vi "test3-SyncMessage_API.vi"(8 "error in (no error)":errorcluster, 11 "TestCase in":refnum<class "testcase-CSMMessage.lvclass">) -> (0 "error out":errorcluster, 3 "TestCase out":refnum<class "testcase-CSMMessage.lvclass">)   [LabVIEW 2017, in "testcase-CSMMessage.lvclass"]
uses:
  testcase-CSMMessage.lvclass
  31aab9b4-27f2-4601-9b9c-9d12425ab602.vi
  src/user.lib/_NEVSTOP/Communicable State Machine(CSM)/AdvanceAPI/CSM - Make String Arguments Safe.vi
  src/user.lib/_NEVSTOP/Communicable State Machine(CSM)/AdvanceAPI/CSM - Keywords.vi
  <vilib>/addons/_JKI Toolkits/VI Tester/TestCase.llb/TestCase.lvclass
  src/user.lib/_NEVSTOP/Communicable State Machine(CSM)/Communicable State Machine.lvlib
  C:/Program Files (x86)/National Instruments/LabVIEW 2017/vi.lib/addons/_JKI Toolkits/VI Tester/TestCase.llb/TestCase.lvclass
panel:
  out "Attribute":T1(array[cluster])
  out "Found":bool[](array[boolean])
  out "Loopcount":i32
  out "concatenated string":string
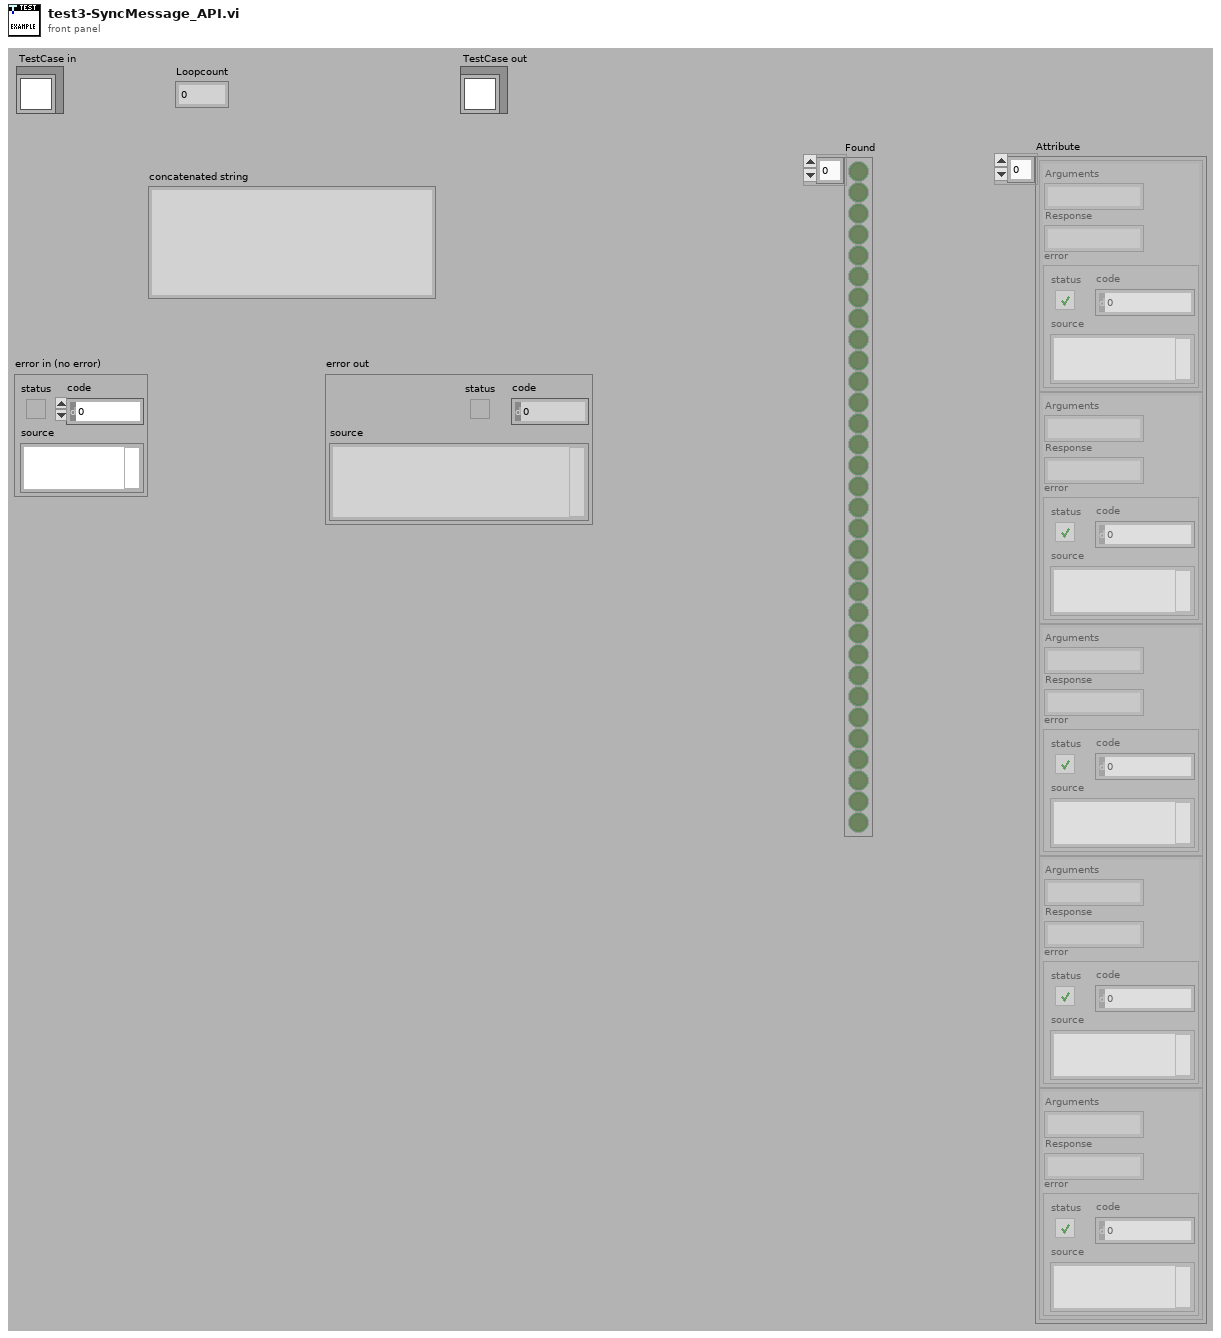
[diagram p1: front panel]
types:
  T1 = cluster{"Arguments":string, "Response":string, "error":errorcluster}[]
  T2 = cluster{"Arguments":string, "Response":string, "error":errorcluster}
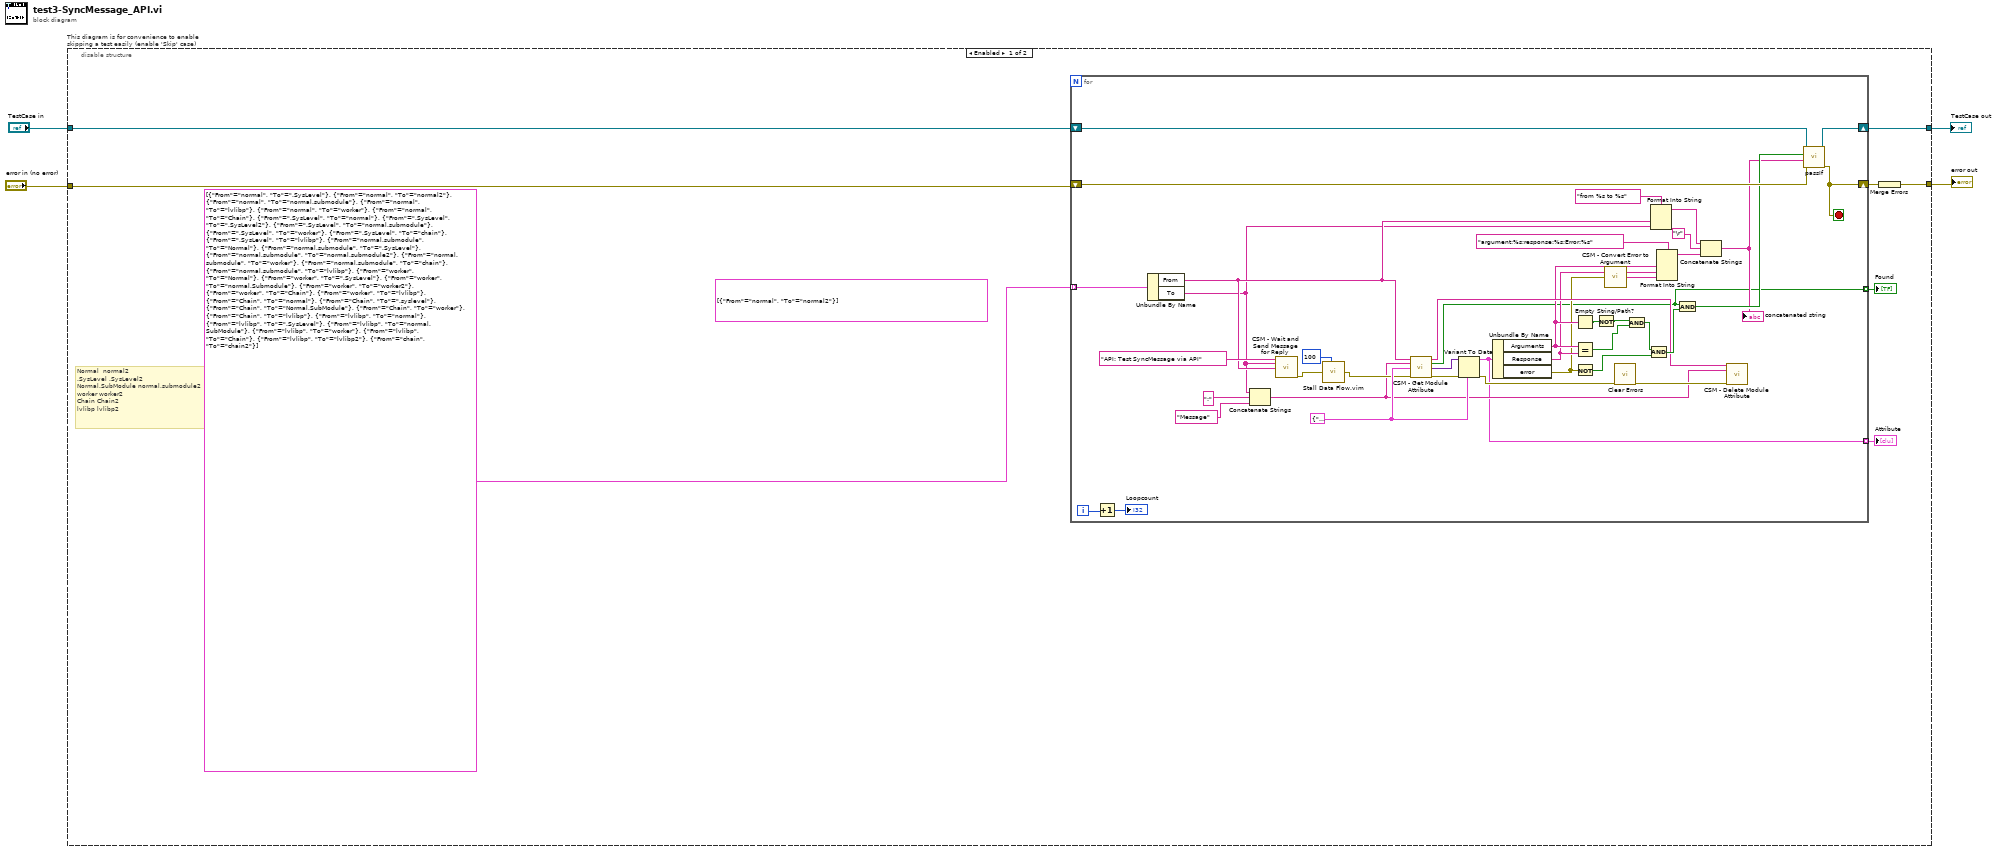
[diagram p0: block diagram]
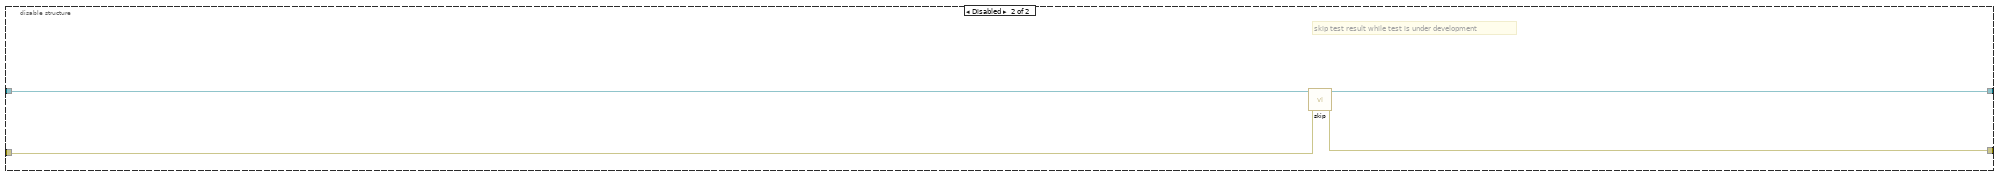
[diagram p2: hidden frame]
diagram:
  n1 = disable-structure "This diagram is for convenience to enable skipping a test easily (enable 'Skip' case)" shown="Enabled" {
    disable-tunnel: "TestCase in" -> [w12 w57]
    disable-tunnel: [w11 w55] -> w1
    disable-tunnel: [w8 w56] -> w3
    disable-tunnel: "error in (no error)" -> [w9 w54]
    frame Enabled {
      (unwired) cluster{"From":string, "To":string}[] [{"From"="normal", "To"="normal2"}]
      # "Normal  normal2\n.SysLevel .SysLevel2\nNormal.SubModule normal.submodule2\nworker worker2\nChain Chain2\nlvlibp lvlibp2"
      n2 = for {
        tunnel: cluster{"From":string, "To":string}[] [{"From"="normal", "To"=".SysLevel"}, {"From"="normal", "To"="normal2"}, {"From"="normal", "To"="normal.submodule"}, {"From"="normal", "To"="lvlibp"}, {"From"="normal", "To"="worker"}, {"From"="normal", "To"="Chain"}, {"From"=".SysLevel", "To"="normal"}, {"From"=".SysLevel", "To"=".SysLevel2"}, {"From"=".SysLevel", "To"="normal.submodule"}, {"From"=".SysLevel", "To"="worker"}, {"From"=".SysLevel", "To"="chain"}, {"From"=".SysLevel", "To"="lvlibp"}, {"From"="normal.submodule", "To"="Normal"}, {"From"="normal.submodule", "To"=".SysLevel"}, {"From"="normal.submodule", "To"="normal.submodule2"}, {"From"="normal.submodule", "To"="worker"}, {"From"="normal.submodule", "To"="chain"}, {"From"="normal.submodule", "To"="lvlibp"}, {"From"="worker", "To"="Normal"}, {"From"="worker", "To"=".SysLevel"}, {"From"="worker", "To"="normal.Submodule"}, {"From"="worker", "To"="worker2"}, {"From"="worker", "To"="Chain"}, {"From"="worker", "To"="lvlibp"}, {"From"="Chain", "To"="normal"}, {"From"="Chain", "To"=".syslevel"}, {"From"="Chain", "To"="Normal.SubModule"}, {"From"="Chain", "To"="worker"}, {"From"="Chain", "To"="lvlibp"}, {"From"="lvlibp", "To"="normal"}, {"From"="lvlibp", "To"=".SysLevel"}, {"From"="lvlibp", "To"="normal.SubModule"}, {"From"="lvlibp", "To"="worker"}, {"From"="lvlibp", "To"="Chain"}, {"From"="lvlibp", "To"="lvlibp2"}, {"From"="chain", "To"="chain2"}] -> [w44] mode=indexing
        shift-right: [w52] -> w11
        shift-left: w12 -> [w53]
        shift-right: [w25] -> w10
        shift-left: w9 -> [w51]
        tunnel: [w16] -> w6 mode=indexing
        tunnel: [w15] -> w5 mode=indexing
        i -> [w18]
        stop <- w25 stop-if-true
        w48 = T2 {"Arguments"="", "Response"="", "error"={"status"=FALSE, "code"=0, "source"=""}}
        n3 = Increment(x=w18) -> (x+1=→"Loopcount":i32)
        n4 = Unbundle By Name(w44) -> ("From"=w22:string, "To"=w20:string)
        n5 = Concatenate Strings(w20, ":" ("string"), "Message" ("string")) -> (w21:string)
        n6 = call "CSM - Wait and Send Message for Reply.vi"("State"="API: Test SyncMessage via API", "Arguments (\"\")"=w20, "Target Module"=w22) -> ("error out"=w14:errorcluster)  [unwired: 9 in, 3 out]
        n7 = call "Stall Data Flow.vim"("value in"=w14, "milliseconds to wait"=u32 100) -> ("value out"=w31:errorcluster)  [unwired: 1 out]
        n8 = call "CSM - Get Module Attribute.vi"("CSM Name"=w22, "Attribute"=w21, "Default Value (Empty Variant)"=w48, "Error In"=w31) -> ("CSM Name (Dup)"=w42:string, "Found"=w16:bool, "Value"=w19:variant, "error out"=w49:errorcluster)  [unwired: 7 in, 1 out]
        n9 = Variant To Data(error in=w49, type=w48, Variant=w19) -> (data=w15:T2, error out=w27:errorcluster)
        n10 = Unbundle By Name(w15) -> ("Arguments"=w37:string, "Response"=w36:string, "error"=w34:errorcluster)
        n11 = Empty String/Path?(string/path=w37) -> (empty?=w41:bool)
        n12 = Equal?(x=w37, y=w36) -> (x = y?=w39:bool)
        n13 = Not(x=w34) -> (.not. x?=w47:bool)
        n14 = Not(x=w41) -> (.not. x?=w40:bool)
        n15 = call "CSM - Convert Error to Argument.vi"("Error"=w34) -> ("Argument"=w35:string)  [unwired: 4 in]
        n16 = call <vilib>:"Clear Errors.vi"("error in (no error)"=w27) -> ("error out"=w26:errorcluster)  [unwired: 5 in, 1 out]
        n17 = And(x=w40, y=w39) -> (x .and. y?=w38:bool)
        n18 = And(x=w38, y=w47) -> (x .and. y?=w46:bool)
        n19 = Format Into String(format string="from %s to %s", w22, w20) -> (resulting string=w29:string)  [unwired: 2 in, 1 out]
        n20 = Format Into String(format string="argument:%s;response:%s;Error:%s", w37, w36, w35) -> (resulting string=w33:string)  [unwired: 2 in, 1 out]
        n21 = And(x=w16, y=w46) -> (x .and. y?=w45:bool)
        n22 = Concatenate Strings(w29, "\r", w33) -> (w30:string)
        "concatenated string" <- w30
        n23 = call "CSM - Delete Module Attribute.vi"("CSM Name"=w42, "Attribute"=w21, "Error In"=w26) -> ()  [unwired: 9 in, 4 out]
        n24 = call-dynamic "passIf.vi"("error in (no error)"=w51, "message (\"\")"=w30, "pass"=w45, "TestCase in"=w53) -> ("error out"=w25:errorcluster, "TestCase out"=w52:refnum<class "testcase-CSMMessage.lvclass">)  [unwired: 6 in]
      }
      "Found" <- w6
      "Attribute" <- w5
      n25 = Merge Errors(w10) -> (w8:errorcluster)
    }
    frame Disabled {
      # "skip test result while test is under development"
      n26 = call <vilib>:"skip.vi"("error in (no error)"=w54, "TestCase in"=w57) -> ("error out"=w56:errorcluster, "TestCase out"=w55:refnum<class "testcase-CSMMessage.lvclass">)  [unwired: 8 in]
    }
  }
  "error out" <- w3
  "TestCase out" <- w1
